vi "SaveData.vi"(8 "error in (no error)":errorcluster, 10 "TDMS File Path":path, 11 "Task_Abstr in":refnum<class "Task_Abstr.lvclass">) -> (0 "error out":errorcluster, 3 "Task_Abstr out":refnum<class "Task_Abstr.lvclass">)   [LabVIEW 2025, in "Task_Abstr.lvlib" / "Task_Abstr.lvclass"]
uses:
  Task_Abstr.lvclass
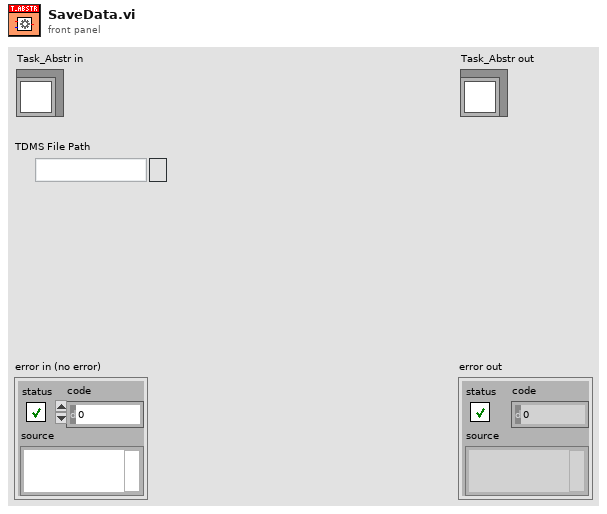
[diagram p1: front panel]
types:
  T1 = enum16{"open", "open or create", "create or replace", "create", "open (read-only)"}
  T2 = typedef "Task_Abstr.lvlib/Task_Abstr.lvclass/DataContainer.ctl" = map{string, T3}
  T3 = typedef "Task_Abstr.lvlib/Task_Abstr.lvclass/WaveformData.ctl" = cluster{"StartTime":timestamp, "StopTime":timestamp, "Waveform":waveform(dbl)[]}
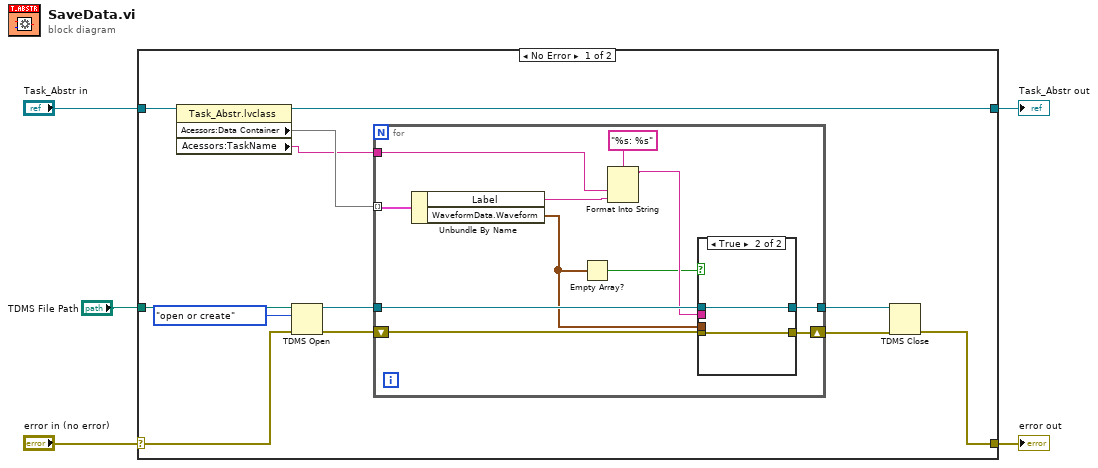
[diagram p0: block diagram]
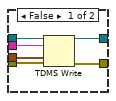
[diagram p2: hidden frame]
diagram:
  n1 = case shown="No Error" "error in (no error)" {
    selector: "error in (no error)" -> [w8 w38]
    tunnel: [w7 w38] -> w4
    tunnel: [w16 w37] -> w2
    tunnel: "Task_Abstr in" -> [w17 w37]
    tunnel: "TDMS File Path" -> [w14 _]
    frame No Error {
      n2 = property class="Task_Abstr.lvclass"(reference=w17) -> (reference out=w16:refnum<class "Task_Abstr.lvclass">, "Acessors:Data Container"=w15:T2, "Acessors:TaskName"=w6:string)  [unwired: 1 in, 1 out]
      n3 = TDMS Open(8:w8, 10:T1."open or create" ("operation (0:open)"), 11:w14) -> (0:w10:errorcluster, 3:w12:refnum<k34>)  [unwired: 4 in]
      n4 = for {
        tunnel: w15 -> [w28] mode=indexing
        tunnel: w12 -> [w27]
        tunnel: [w26] -> w11
        shift-right: [w24] -> w9
        shift-left: w10 -> [w25]
        tunnel: w6 -> [w22]
        n5 = Unbundle By Name(w28) -> ("Label"=w21:string, "WaveformData.Waveform"=w19:waveform(dbl)[])
        n6 = Empty Array?(array=w19) -> (empty?=w18:bool)
        n7 = Format Into String(format string="%s: %s", w22, w21) -> (resulting string=w20:string)  [unwired: 2 in, 1 out]
        n8 = case shown="True" w18 {
          tunnel: w27 -> [w34 w36]
          tunnel: [w33 w36] -> w26
          tunnel: w25 -> [w32 w35]
          tunnel: [w31 w35] -> w24
          tunnel: w20 -> [w30 _]
          tunnel: w19 -> [w29 _]
          frame False {
            n9 = TDMS Write(0:w34, 5:w30, 9:w29, 11:w32) -> (4:w33:refnum<k34>, 15:w31:errorcluster)  [unwired: 2 in, 2 out]
          }
          frame True {
          }
        }
      }
      n10 = TDMS Close(8:w9, 11:w11) -> (0:w7:errorcluster)  [unwired: 1 out]
    }
    frame Error {
    }
  }
  "error out" <- w4
  "Task_Abstr out" <- w2
